vi "Get Work Area and Display Mode(冲突时的文件备份2013-03-27 14-08-24).vi"(8 "错误输入（无错误）":errorcluster) -> (0 "错误输出":errorcluster, 2 "显示:主工作区":T2, 3 "显示分辨率":T1)   [LabVIEW 2012, in "Application.lvlib"]
uses:
  Application.lvlib
  <vilib>/Utility/miscctls.llb/LVRectTypeDef.ctl
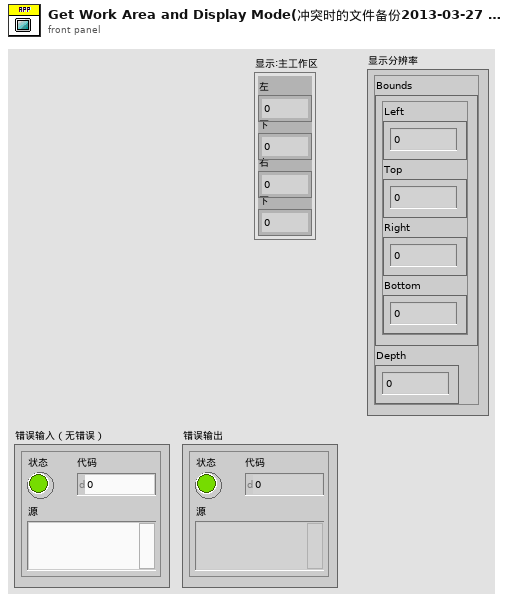
[diagram p1: front panel]
types:
  T1 = cluster{"Bounds":cluster{"Left":i16, "Top":i16, "Right":i16, "Bottom":i16}, "Depth":i16}
  T2 = typedef "LVRectTypeDef.ctl" = cluster{"Left":i16, "Top":i16, "Right":i16, "Bottom":i16}
  T3 = typedef "LVAllMonitorsDisplayTypeDef.ctl" = cluster{"Bounds":cluster{"Left":i16, "Top":i16, "Right":i16, "Bottom":i16}, "Depth":i16}[]
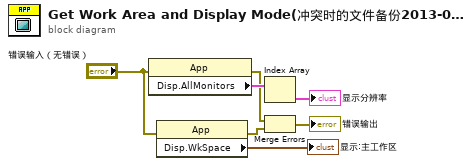
[diagram p0: block diagram]
diagram:
  n1 = property class="App"(error in="错误输入（无错误）") -> (error out=w3:errorcluster, "Disp.AllMonitors"=w6:T3)  [unwired: 1 in, 1 out]
  n2 = property class="App"(error in="错误输入（无错误）") -> (error out=w2:errorcluster, "Disp.WkSpace"=→"显示:主工作区":T2)  [unwired: 1 in, 1 out]
  n3 = Index Array(array=w6) -> (element=→"显示分辨率":T1)  [unwired: 1 in]
  n4 = Merge Errors(w3, w2) -> (→"错误输出":errorcluster)
